vi "Hall Effect Test.vi"(8 "error in (no error)":errorcluster) -> (0 "error out":errorcluster)   [LabVIEW 2016, in "Hall Effect Library.lvlib"]
uses:
  Hall Effect Library.lvlib
  Controls/Measurement.ctl
  Public/Controls/Data Items.ctl
  Public/Controls/Tests.ctl
  Global Variables/Hall Effect Data.vi
  Global Variables/Test Settings.vi
  Global Variables/Instrument Locations.vi
panel:
  out "Test Step":T1(ring)
  out "Measurement":T2
  out "Soak Until":timestamp
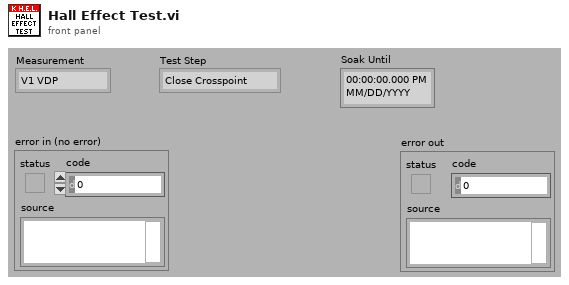
[diagram p1: front panel]
types:
  T1 = enum16{"Close Crosspoint", "Soak 1", "Zero Ammeter", "Zero Voltmeter", "I-SRC On", "Init Ammeter", "Soak 2", "Measure I", "Measure V", "I-SRC Off", "Open Crosspoint", "Done"}
  T2 = typedef "Hall Effect Library.lvlib/Measurement.ctl" = enum16{"V1 VDP", "V2 VDP", "V3 VDP", "V4 VDP", "V5 VDP", "V6 VDP", "V7 VDP", "V8 VDP", "V1 HE", "V2 HE", "V3 HE", "V4 HE", "V5 HE", "V6 HE", "V7 HE", "V8 HE", "V1 Res Bar", "V1 Hall Bar", "V1 Res 6-Cot", "V2 Res 6-Cot", "V3 Res 6-Cot", "V4 Res 6-Cot", "V1 Hall 6-Cot", "V2 Hall 6-Cot", "V3 Hall 6-Cot", "V4 Hall 6-Cot", "V5 Hall 6-Cot", "V6 Hall 6-Cot", "V7 Hall 6-Cot", "V8 Hall 6-Cot", "V1 Res 8-Cot", "V2 Res 8-Cot", "V3 Res 8-Cot", "V4 Res 8-Cot", "V1 Hall 8-Cot", "V2 Hall 8-Cot", "V3 Hall 8-Cot", "V4 Hall 8-Cot"}
  T3 = cluster{"RHD":dbl, "RHC":dbl, "RHAvg":dbl, "uH":dbl, "n/p":dbl}
  T4 = typedef "Hall Effect Library.lvlib/Resisitivity.ctl" = enum16{"Low", "High"}
  T5 = typedef "Hall Effect Library.lvlib/Tests.ctl" = enum16{"Van Der Pauw", "Hall Effect", "Bar Sample Resistivity", "Bar Sample Hall ", "6-Contact Sample Resistivity", "6-Contact Sample Hall", "8-Contact Sample Resistivity", "8-Contact Sample Hall", ""}
  T6 = typedef "Hall Effect Library.lvlib/Data Items.ctl" = enum16{"V1 Van Der Pauw", "V2 Van Der Pauw", "V3 Van Der Pauw", "V4 Van Der Pauw", "V5 Van Der Pauw", "V6 Van Der Pauw", "V7 Van Der Pauw", "V8 Van Der Pauw", "V1 Hall Effect", "V2 Hall Effect", "V3 Hall Effect", "V4 Hall Effect", "V5 Hall Effect", "V6  Hall Effect", "V7 Hall Effect", "V8 Hall Effect", "V1 Res Bar", "V1 Hall Bar", "V1 Res 6-Cot", "V2 Res 6-Cot", "V3 Res 6-Cot", "V4 Res 6-Cot", "V1 Hall 6-Cot", "V2 Hall 6-Cot", "V3 Hall 6-Cot", "V4 Hall 6-Cot", "V5 Hall 6-Cot", "V6 Hall 6-Cot", "V7 Hall 6-Cot", "V8 Hall 6-Cot", "V1 Res 8-Cot", "V2 Res 8-Cot", "V3 Res 8-Cot", "V4 Res 8-Cot", "V1 Hall 8-Cot", "V2 Hall 8-Cot", "V3 Hall 8-Cot", "V4 Hall 8-Cot", "Van Der Pauw Results", "Hall Effect Results", "Bar Sample Resistivity Results", "Bar Sample Hall Results", "6-Contact Resistivity Results", "6-Contact Hall Results", "8-Contact Resistivity Results", "8-Contact Hall Results"}
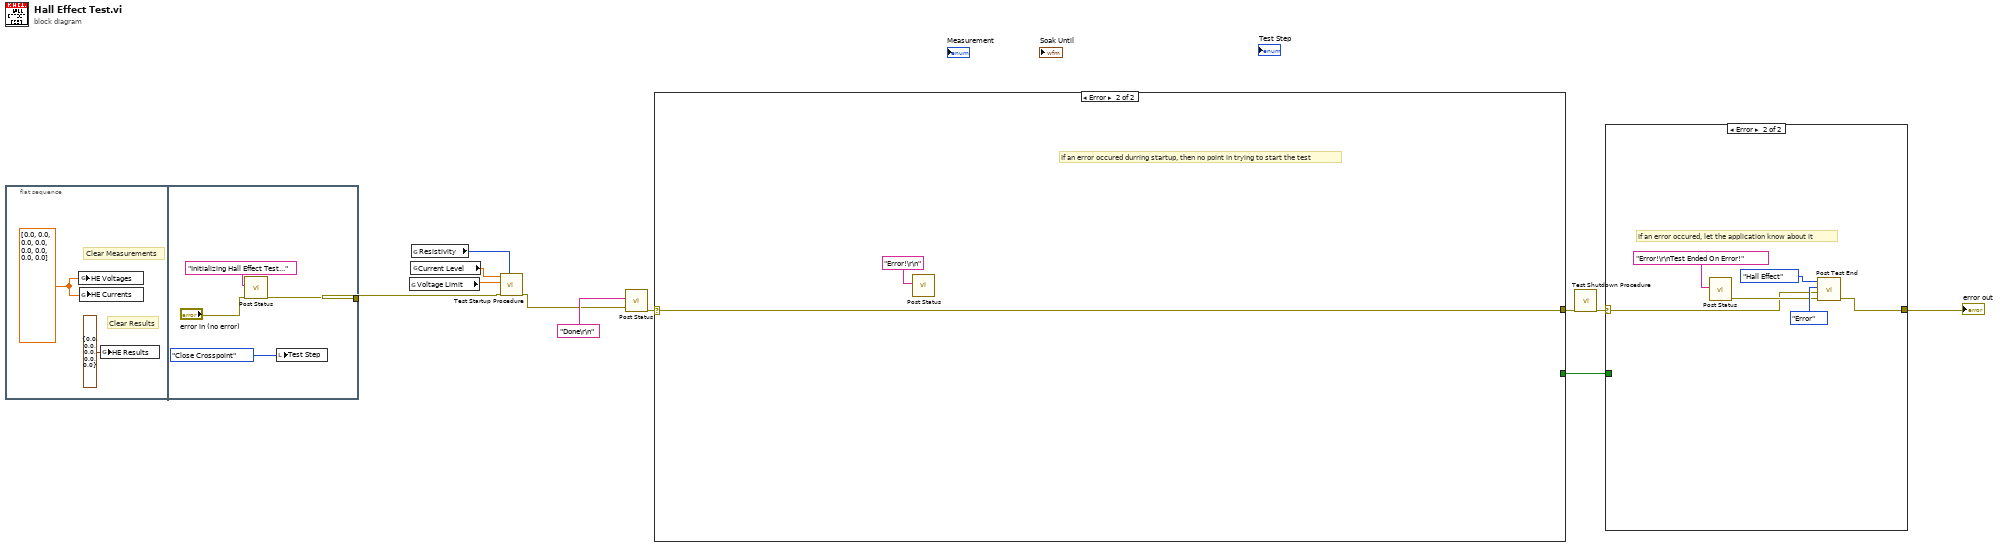
[diagram p0: block diagram]
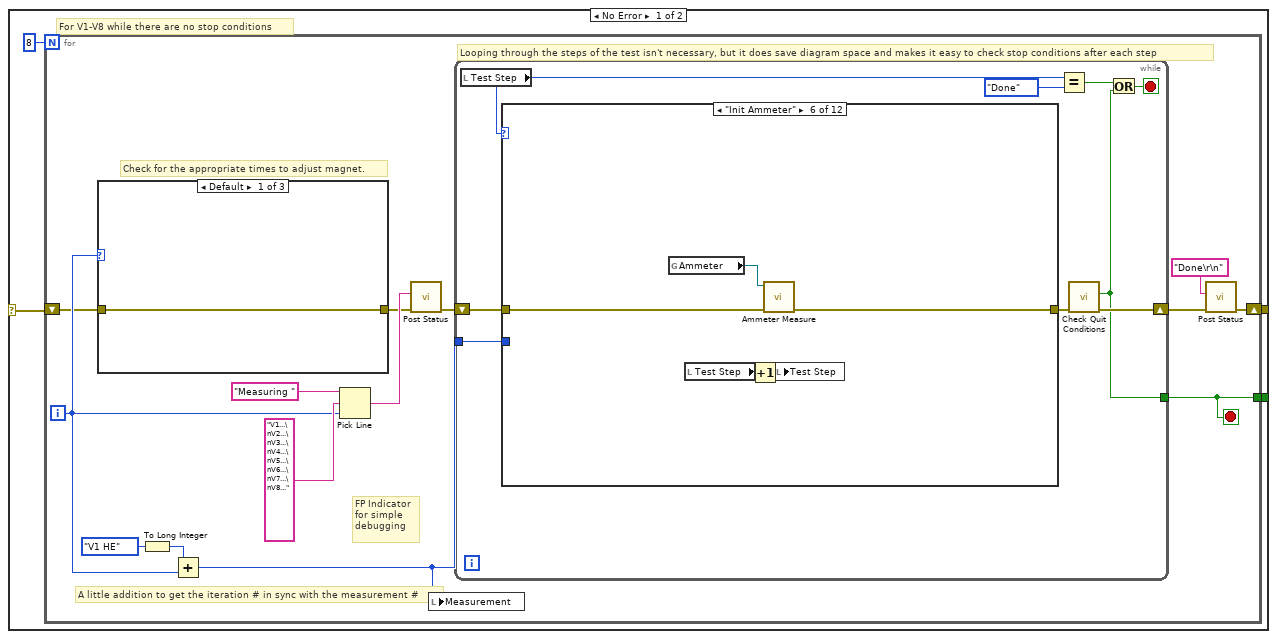
[diagram p2: hidden frame]
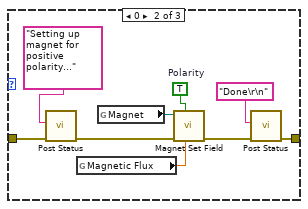
[diagram p3: hidden frame]
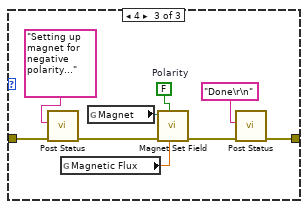
[diagram p4: hidden frame]
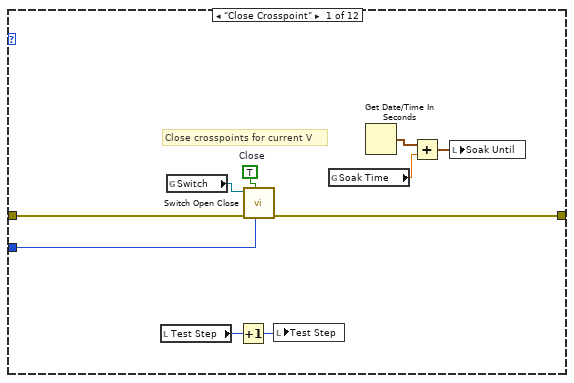
[diagram p5: hidden frame]
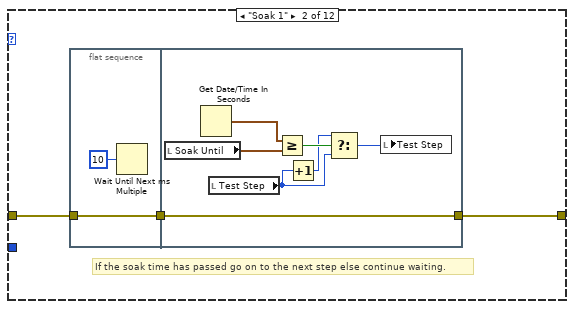
[diagram p6: hidden frame]
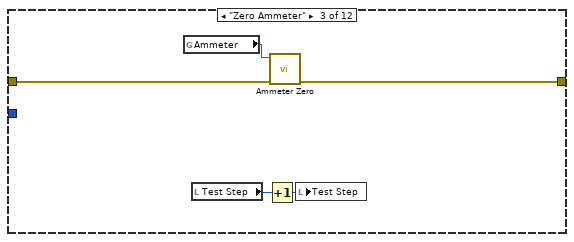
[diagram p7: hidden frame]
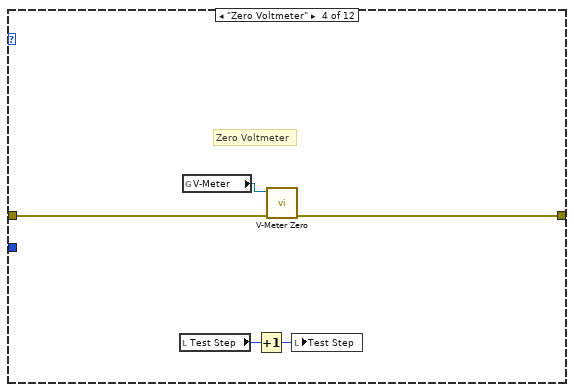
[diagram p8: hidden frame]
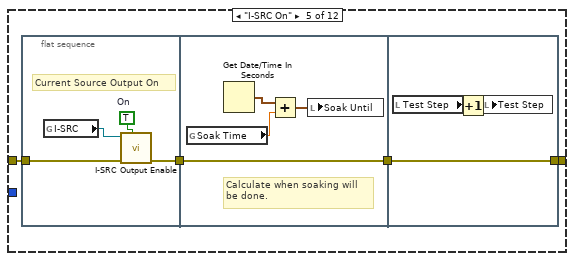
[diagram p9: hidden frame]
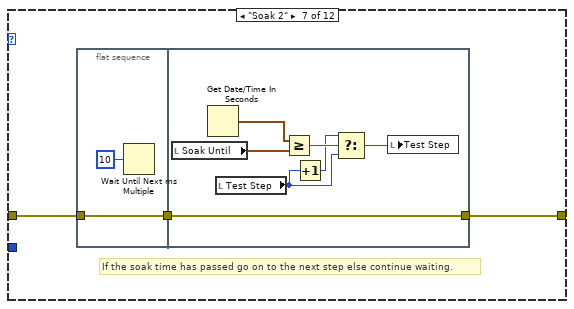
[diagram p10: hidden frame]
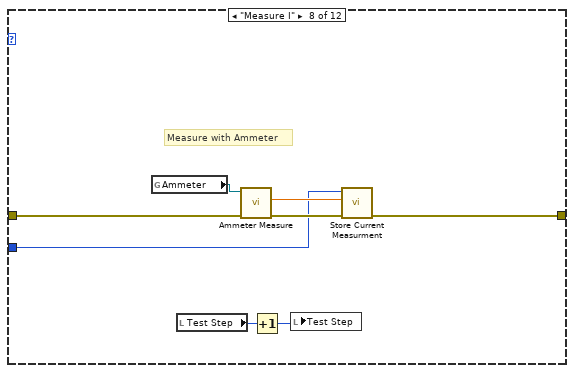
[diagram p11: hidden frame]
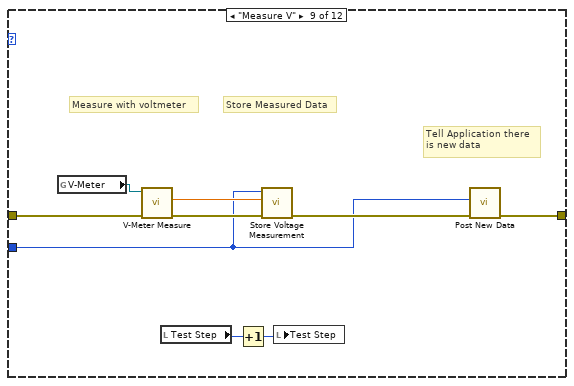
[diagram p12: hidden frame]
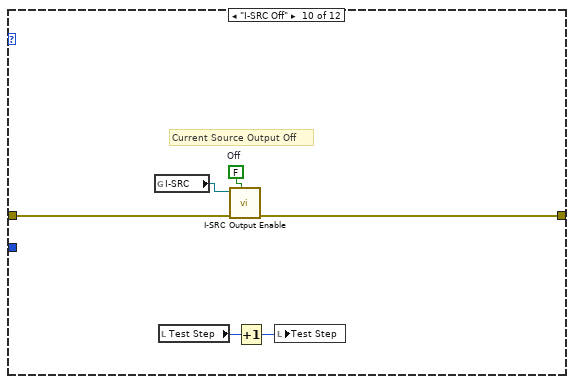
[diagram p13: hidden frame]
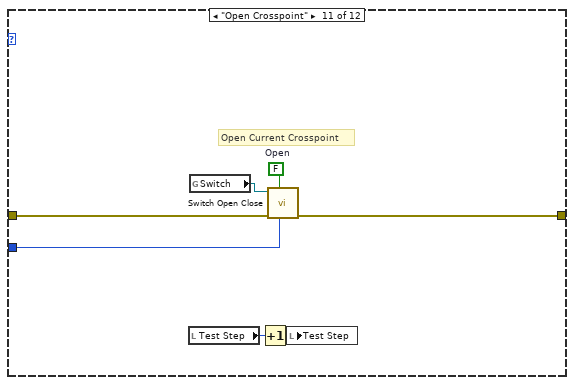
[diagram p14: hidden frame]
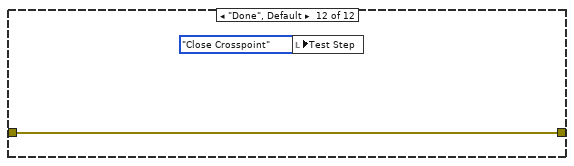
[diagram p15: hidden frame]
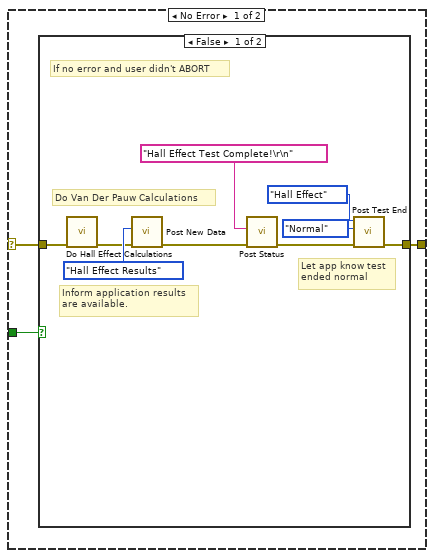
[diagram p16: hidden frame]
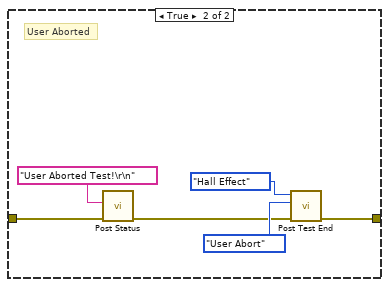
[diagram p17: hidden frame]
diagram:
  n1 = flat-sequence {
    tunnel: [w14] -> w2
    frame #0 {
      w13 = dbl[] [0.0, 0.0, 0.0, 0.0, 0.0, 0.0, 0.0, 0.0] ("Van Der Pauw Voltages")
      # "Clear Results"
      # "Clear Measurements"
      n2 = global write "Hall Effect Data.vi" "HE Voltages"(w13) -> ()
      n3 = global write "Hall Effect Data.vi" "HE Currents"(w13) -> ()
      n4 = global write "Hall Effect Data.vi" "HE Results"(T3 {"RHD"=0.0, "RHC"=0.0, "RHAvg"=0.0, "uH"=0.0, "n/p"=0.0} ("HE Results")) -> ()
    }
    frame #1 {
      n5 = call "Post Status.vi"("error in (no error)"="error in (no error)", "Status Message"="Initializing Hall Effect Test...") -> ("error out"=w14:errorcluster)  [unwired: 9 out]
      n6 = local write "Test Step"(T1."Close Crosspoint" ("Test Step")) -> ()
    }
  }
  n7 = global read "Test Settings.vi" "Voltage Limit"() -> (w3:dbl)
  n8 = global read "Test Settings.vi" "Current Level"() -> (w4:dbl)
  n9 = global read "Test Settings.vi" "Resistivity"() -> (w5:T4)
  n10 = call "Test Startup Procedure.vi"("Resistivity"=w5, "error in (no error)"=w2, "Voltage Limit"=w3, "Current Level"=w4) -> ("error out"=w1:errorcluster)  [unwired: 7 out]
  n11 = call "Post Status.vi"("error in (no error)"=w1, "Status Message"="Done\r\n") -> ("error out"=w9:errorcluster)  [unwired: 9 out]
  n12 = case shown="Error" w9 {
    selector: w9 -> [w19 w161]
    tunnel: [w21 w161] -> w7
    tunnel: [w20 _] -> w10
    frame No Error {
      # "For V1-V8 while there are no stop conditions"
      n13 = for {
        N: 8 -> [_]
        shift-right: [w25] -> w21
        shift-left: w19 -> [w27]
        tunnel: [w22] -> w20
        i -> [w29]
        stop <- w22 stop-if-true
        # "A little addition to get the iteration # in sync with the measurement #"
        # "Check for the appropriate times to adjust magnet."
        # "FP Indicator\nfor simple\ndebugging"
        # "Looping through the steps of the test isn't necessary, but it does save diagram space and makes it easy to check stop conditions after each step"
        n14 = case shown="Default" w29 {
          tunnel: [w36 w39 w47] -> w28
          tunnel: w27 -> [w36 w42 w51]
          frame Default {
          }
          frame 0 {
            w43 = TRUE  # Polarity
            n15 = call "Post Status.vi"("error in (no error)"=w42, "Status Message"="Setting up magnet for positive polarity...") -> ("error out"=w41:errorcluster)  [unwired: 9 out]
            n16 = global read "Test Settings.vi" "Magnetic Flux"() -> (w45:dbl)
            n17 = global read "Instrument Locations.vi" "Magnet"() -> (w44:refnum<visa-resource-name>)
            n18 = call "Magnet Set Field.vi"("Field Strength"=w45, "Polarity"=w43, "error in (no error)"=w41, "VISA resource name in"=w44) -> ("error out"=w40:errorcluster)  [unwired: 7 out]
            n19 = call "Post Status.vi"("error in (no error)"=w40, "Status Message"="Done\r\n") -> ("error out"=w39:errorcluster)  [unwired: 9 out]
          }
          frame 4 {
            w52 = FALSE  # Polarity
            n20 = call "Post Status.vi"("error in (no error)"=w51, "Status Message"="Setting up magnet for negative polarity...") -> ("error out"=w50:errorcluster)  [unwired: 9 out]
            n21 = global read "Test Settings.vi" "Magnetic Flux"() -> (w54:dbl)
            n22 = global read "Instrument Locations.vi" "Magnet"() -> (w53:refnum<visa-resource-name>)
            n23 = call "Magnet Set Field.vi"("Field Strength"=w54, "Polarity"=w52, "error in (no error)"=w50, "VISA resource name in"=w53) -> ("error out"=w48:errorcluster)  [unwired: 7 out]
            n24 = call "Post Status.vi"("error in (no error)"=w48, "Status Message"="Done\r\n") -> ("error out"=w47:errorcluster)  [unwired: 9 out]
          }
        }
        n25 = To Long Integer(number=Measurement."V1 HE" ("Measurement")) -> (32bit integer=w31:i32)
        n26 = Add(x=w31, y=w29) -> (x+y=w23:i32)
        n27 = Pick Line(string ("")="Measuring ", multi-line string="V1...\nV2...\nV3...\nV4...\nV5...\nV6...\nV7...\nV8...", line index=w29) -> (output string=w33:string)
        n28 = call "Post Status.vi"("error in (no error)"=w28, "Status Message"=w33) -> ("error out"=w32:errorcluster)  [unwired: 9 out]
        n29 = local write "Measurement"(w23) -> ()
        n30 = while {
          shift-right: [w61] -> w24
          shift-left: w32 -> [w63]
          tunnel: w23 -> [w62]
          tunnel: [w57] -> w22
          stop <- w60 stop-if-true
          n31 = local read "Test Step"() -> (w58:T1)
          n32 = case shown="\"Init Ammeter\"" w58 {
            tunnel: [w71 w74 w89 w93 w98 w114 w117 w132 w139 w147 w155 w159] -> w56
            tunnel: w63 -> [w70 w75 w90 w94 w99 w115 w118 w134 w143 w148 w154 w159]
            tunnel: w62 -> [w69 _ _ _ _ _ _ w130 w138 _ w153 _]
            frame "Close Crosspoint" {
              w72 = TRUE  # Close
              # "Close crosspoints for current V"
              n33 = local read "Test Step"() -> (w67:T1)
              n34 = global read "Instrument Locations.vi" "Switch"() -> (w73:refnum<visa-resource-name>)
              n35 = Increment(x=w67) -> (x+1=w68:T1)
              n36 = call "Switch Open Close.vi"("Measurement"=w69, "Open/Close (F: Open)"=w72, "error in (no error)"=w70, "VISA resource name in"=w73) -> ("error out"=w71:errorcluster)  [unwired: 7 out]
              n37 = local write "Test Step"(w68) -> ()
              n38 = global read "Test Settings.vi" "Soak Time"() -> (w65:dbl)
              n39 = Get Date/Time In Seconds() -> (seconds since 1Jan1904=w64:timestamp)
              n40 = Add(x=w64, y=w65) -> (x+y=w66:timestamp)
              n41 = local write "Soak Until"(w66) -> ()
            }
            frame "Soak 1" {
              # "If the soak time has passed go on to the next step else continue waiting."
              n42 = flat-sequence {
                tunnel: w75 -> [w77]
                tunnel: [w77] -> w76
                tunnel: [w81] -> w74
                tunnel: w76 -> [w81]
                frame #0 {
                  n43 = Wait Until Next ms Multiple(millisecond multiple=u32 10) -> ()  [unwired: 1 out]
                }
                frame #1 {
                  n44 = local read "Soak Until"() -> (w84:timestamp)
                  n45 = Get Date/Time In Seconds() -> (seconds since 1Jan1904=w85:timestamp)
                  n46 = local read "Test Step"() -> (w79:T1)
                  n47 = Greater Or Equal?(x=w85, y=w84) -> (x >= y?=w83:bool)
                  n48 = Increment(x=w79) -> (x+1=w80:T1)
                  n49 = Select(t=w80, s=w83, f=w79) -> (s? t:f=w82:T1)
                  n50 = local write "Test Step"(w82) -> ()
                }
              }
            }
            frame "Zero Ammeter" {
              n51 = global read "Instrument Locations.vi" "Ammeter"() -> (w88:refnum<visa-resource-name>)
              n52 = local read "Test Step"() -> (w86:T1)
              n53 = Increment(x=w86) -> (x+1=w87:T1)
              n54 = call "Ammeter Zero.vi"("error in (no error)"=w90, "VISA resource name in"=w88) -> ("error out"=w89:errorcluster)  [unwired: 9 out]
              n55 = local write "Test Step"(w87) -> ()
            }
            frame "Zero Voltmeter" {
              # "Zero Voltmeter"
              n56 = local read "Test Step"() -> (w92:T1)
              n57 = global read "Instrument Locations.vi" "V-Meter"() -> (w95:refnum<visa-resource-name>)
              n58 = Increment(x=w92) -> (x+1=w91:T1)
              n59 = call "V-Meter Zero.vi"("error in (no error)"=w94, "VISA resource name in"=w95) -> ("error out"=w93:errorcluster)  [unwired: 9 out]
              n60 = local write "Test Step"(w91) -> ()
            }
            frame "I-SRC On" {
              n61 = flat-sequence {
                tunnel: w99 -> [w101]
                tunnel: [w100] -> w97
                tunnel: w97 -> [w107]
                tunnel: [w107] -> w96
                tunnel: [w110] -> w98
                tunnel: w96 -> [w110]
                frame #0 {
                  w102 = TRUE  # On
                  # "Current Source Output On"
                  n62 = global read "Instrument Locations.vi" "I-SRC"() -> (w103:refnum<visa-resource-name>)
                  n63 = call "I-SRC Output Enable.vi"("Output (Off)"=w102, "error in (no error)"=w101, "VISA resource name in"=w103) -> ("error out"=w100:errorcluster)  [unwired: 8 out]
                }
                frame #1 {
                  # "Calculate when soaking will\nbe done."
                  n64 = global read "Test Settings.vi" "Soak Time"() -> (w105:dbl)
                  n65 = Get Date/Time In Seconds() -> (seconds since 1Jan1904=w104:timestamp)
                  n66 = Add(x=w104, y=w105) -> (x+y=w106:timestamp)
                  n67 = local write "Soak Until"(w106) -> ()
                }
                frame #2 {
                  n68 = local read "Test Step"() -> (w109:T1)
                  n69 = Increment(x=w109) -> (x+1=w108:T1)
                  n70 = local write "Test Step"(w108) -> ()
                }
              }
            }
            frame "Init Ammeter" {
              n71 = global read "Instrument Locations.vi" "Ammeter"() -> (w113:refnum<visa-resource-name>)
              n72 = local read "Test Step"() -> (w112:T1)
              n73 = Increment(x=w112) -> (x+1=w111:T1)
              n74 = call "Ammeter Measure.vi"("error in (no error)"=w115, "VISA resource name in"=w113) -> ("error out"=w114:errorcluster)  [unwired: 9 out]
              n75 = local write "Test Step"(w111) -> ()
            }
            frame "Soak 2" {
              # "If the soak time has passed go on to the next step else continue waiting."
              n76 = flat-sequence {
                tunnel: w118 -> [w119]
                tunnel: [w119] -> w116
                tunnel: [w123] -> w117
                tunnel: w116 -> [w123]
                frame #0 {
                  n77 = Wait Until Next ms Multiple(millisecond multiple=u32 10) -> ()  [unwired: 1 out]
                }
                frame #1 {
                  n78 = local read "Soak Until"() -> (w126:timestamp)
                  n79 = Get Date/Time In Seconds() -> (seconds since 1Jan1904=w127:timestamp)
                  n80 = local read "Test Step"() -> (w121:T1)
                  n81 = Greater Or Equal?(x=w127, y=w126) -> (x >= y?=w125:bool)
                  n82 = Increment(x=w121) -> (x+1=w122:T1)
                  n83 = Select(t=w122, s=w125, f=w121) -> (s? t:f=w124:T1)
                  n84 = local write "Test Step"(w124) -> ()
                }
              }
            }
            frame "Measure I" {
              # "Measure with Ammeter"
              n85 = global read "Instrument Locations.vi" "Ammeter"() -> (w135:refnum<visa-resource-name>)
              n86 = local read "Test Step"() -> (w129:T1)
              n87 = call "Ammeter Measure.vi"("error in (no error)"=w134, "VISA resource name in"=w135) -> ("error out"=w133:errorcluster, "Measurement"=w131:dbl)  [unwired: 8 out]
              n88 = Increment(x=w129) -> (x+1=w128:T1)
              n89 = local write "Test Step"(w128) -> ()
              n90 = call "Store Current Measurment.vi"("error in"=w133, "Value"=w131, "Measurement"=w130) -> ("error out"=w132:errorcluster)  [unwired: 8 out]
            }
            frame "Measure V" {
              # "Tell Application there\nis new data"
              # "Store Measured Data"
              # "Measure with voltmeter"
              n91 = global read "Instrument Locations.vi" "V-Meter"() -> (w144:refnum<visa-resource-name>)
              n92 = call "V-Meter Measure.vi"("error in (no error)"=w143, "VISA resource name in"=w144) -> ("error out"=w142:errorcluster, "Measurement"=w141:dbl)  [unwired: 1 in, 7 out]
              n93 = local read "Test Step"() -> (w136:T1)
              n94 = Increment(x=w136) -> (x+1=w137:T1)
              n95 = call "Store Voltage Measurement.vi"("error in"=w142, "Value"=w141, "Measurement"=w138) -> ("error out"=w140:errorcluster)  [unwired: 8 out]
              n96 = local write "Test Step"(w137) -> ()
              n97 = call "Post New Data.vi"("error in (no error)"=w140, "Data Item"=w138) -> ("error out"=w139:errorcluster)  [unwired: 9 out]
            }
            frame "I-SRC Off" {
              w149 = FALSE  # Off
              # "Current Source Output Off"
              n98 = global read "Instrument Locations.vi" "I-SRC"() -> (w150:refnum<visa-resource-name>)
              n99 = local read "Test Step"() -> (w146:T1)
              n100 = call "I-SRC Output Enable.vi"("Output (Off)"=w149, "error in (no error)"=w148, "VISA resource name in"=w150) -> ("error out"=w147:errorcluster)  [unwired: 8 out]
              n101 = Increment(x=w146) -> (x+1=w145:T1)
              n102 = local write "Test Step"(w145) -> ()
            }
            frame "Open Crosspoint" {
              w156 = FALSE  # Open
              # "Open Current Crosspoint"
              n103 = local read "Test Step"() -> (w152:T1)
              n104 = global read "Instrument Locations.vi" "Switch"() -> (w157:refnum<visa-resource-name>)
              n105 = Increment(x=w152) -> (x+1=w151:T1)
              n106 = call "Switch Open Close.vi"("Measurement"=w153, "Open/Close (F: Open)"=w156, "error in (no error)"=w154, "VISA resource name in"=w157) -> ("error out"=w155:errorcluster)  [unwired: 7 out]
              n107 = local write "Test Step"(w151) -> ()
            }
            frame "Done", Default {
              n108 = local write "Test Step"(T1."Close Crosspoint" ("Test Step")) -> ()
            }
          }
          n109 = Equal?(x=w58, y=T1."Done") -> (x = y?=w59:bool)
          n110 = call "Check Quit Conditions.vi"("error in (no error)"=w56) -> ("error out"=w61:errorcluster, "Quit?"=w57:bool)  [unwired: 9 out]
          n111 = Or(x=w59, y=w57) -> (x .or. y?=w60:bool)
        }
        n112 = call "Post Status.vi"("error in (no error)"=w24, "Status Message"="Done\r\n") -> ("error out"=w25:errorcluster)  [unwired: 9 out]
      }
    }
    frame Error {
      # "If an error occured durring startup, then no point in trying to start the test"
      n113 = call "Post Status.vi"("Status Message"="Error!\r\n") -> ()  [unwired: 1 in, 10 out]
    }
  }
  n114 = call "Test Shutdown Procedure.vi"("error in (no error)"=w7) -> ("error out"=w6:errorcluster)  [unwired: 10 out]
  n115 = case shown="Error" w6 {
    selector: w6 -> [w163 w181]
    tunnel: w10 -> [w164 _]
    tunnel: [w162 w182] -> w11
    frame No Error {
      n116 = case shown="False" w164 {
        tunnel: w163 -> [w166 w178]
        tunnel: [w168 w175] -> w162
        frame False {
          # "Let app know test\nended normal"
          # "Inform application results\nare available."
          # "Do Van Der Pauw Calculations"
          # "If no error and user didn't ABORT"
          n117 = call "Do Hall Effect Calculations.vi"("error in (no error)"=w166) -> ("error out"=w167:errorcluster)  [unwired: 10 out]
          n118 = call "Post New Data.vi"("error in (no error)"=w167, "Data Item"=Data_Items."Hall Effect Results") -> ("error out"=w171:errorcluster)  [unwired: 9 out]
          n119 = call "Post Status.vi"("error in (no error)"=w171, "Status Message"="Hall Effect Test Complete!\r\n") -> ("error out"=w170:errorcluster)  [unwired: 9 out]
          n120 = call "Post Test End.vi"("error in (no error)"=w170, "Test End"=enum16{"Normal", "User Abort", "Error"}."Normal", "Test"=Tests."Hall Effect") -> ("error out"=w168:errorcluster)  [unwired: 1 in, 7 out]
        }
        frame True {
          # "User Aborted"
          n121 = call "Post Status.vi"("error in (no error)"=w178, "Status Message"="User Aborted Test!\r\n") -> ("error out"=w177:errorcluster)  [unwired: 9 out]
          n122 = call "Post Test End.vi"("error in (no error)"=w177, "Test End"=enum16{"Normal", "User Abort", "Error"}."User Abort", "Test"=Tests."Hall Effect") -> ("error out"=w175:errorcluster)  [unwired: 1 in, 7 out]
        }
      }
    }
    frame Error {
      # "If an error occured, let the application know about it"
      n123 = call "Post Status.vi"("Status Message"="Error!\r\nTest Ended On Error!") -> ("error out"=w184:errorcluster)  [unwired: 1 in, 9 out]
      n124 = call "Post Test End.vi"("error in (no error)"=w184, "Test End Error (no error)"=w181, "Test End"=enum16{"Normal", "User Abort", "Error"}."Error", "Test"=Tests."Hall Effect") -> ("error out"=w182:errorcluster)  [unwired: 7 out]
    }
  }
  "error out" <- w11
